vi "Dialog Macro File Exists Message.vi"(8 "error in (no error)":errorcluster) -> (0 "error out":errorcluster, 3 "Confirmed?":bool)   [LabVIEW 2012]
doc: "SciScan 1.2 160622"
panel:
  in  "Cancel Button":bool
  in  "OK Button":bool
  # "A SciScript file with the name you specified exists!"
  # "Press OK to confirm overwrite\nPress Cancel to abort."
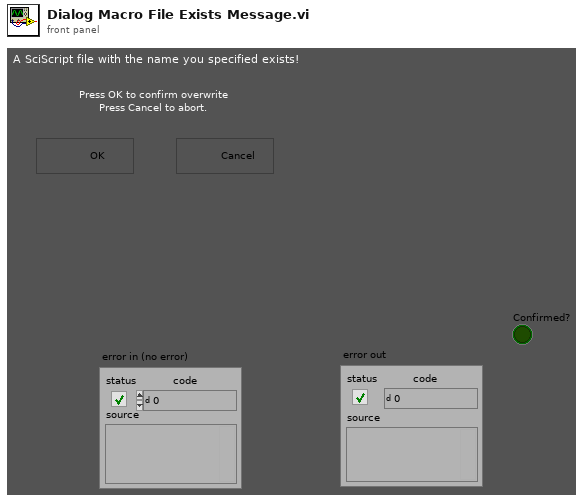
[diagram p1: front panel]
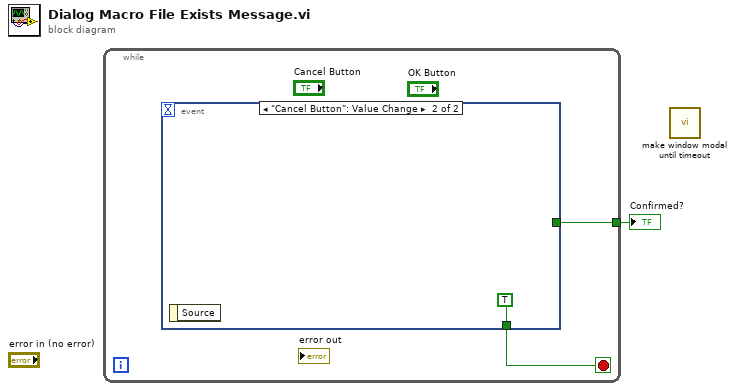
[diagram p0: block diagram]
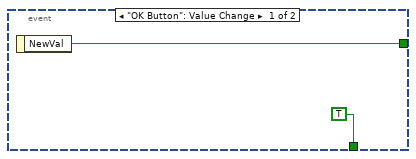
[diagram p2: hidden frame]
diagram:
  n1 = while {
    tunnel: [w3] -> w1
    stop <- w2 stop-if-true
    n2 = event shown="[1] \"Cancel Button\": Value Change" {
      selector: _ -> [_ _]
      dyn-events: _ -> [_ _]
      timeout: _ -> [_ _]
      tunnel: [w4 _] -> w3
      tunnel: [TRUE TRUE] -> w2
      event "OK Button": Value Change {
        n3 = event-data() -> ("NewVal"=w4:bool)  [unwired: 1 in]
      }
      event "Cancel Button": Value Change {
        n4 = event-data() -> ()  [unwired: 1 in, 1 out]
      }
    }
  }
  "Confirmed?" <- w1
  n5 = call "make window modal until timeout.vi"() -> ()  [unwired: 12 in]
